vi "Aeroflex ATT Config Test.vi"(8 "error in (no error)":errorcluster, 10 "Configuration":T2={"BusType"=enum."USB", "Card"=0, "USB"="", "IP"=0, "COM"=1, "Baud Rate"=enum."9600"}, 11 "Str Refnum":refnum<vi>) -> (0 "error out":errorcluster, 3 "Aerolex ATT":T1)   [LabVIEW 2011]
uses:
  TypeDefs/Aeroflex ATT Configuration.ctl
  TypeDefs/Aeroflex ATT Instrument Info.ctl
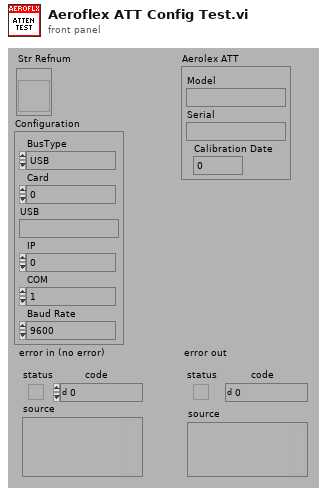
[diagram p1: front panel]
types:
  T1 = typedef "Aeroflex ATT Instrument Info.ctl" = cluster{"Model":string, "Serial":string, "Calibration Date":dbl}
  T2 = typedef "Aeroflex ATT Configuration.ctl" = cluster{"BusType":enum32{"PCI/ISA/PCMCIA", "USB", "Ethernet", "Serial"}, "Card":i32, "USB":string, "IP":u32, "COM":i32, "Baud Rate":enum16{"300", "600", "1200", "2400", "4800", "9600"}}
  T3 = enum32{"PCI/ISA/PCMCIA", "USB", "Ethernet", "Serial"}
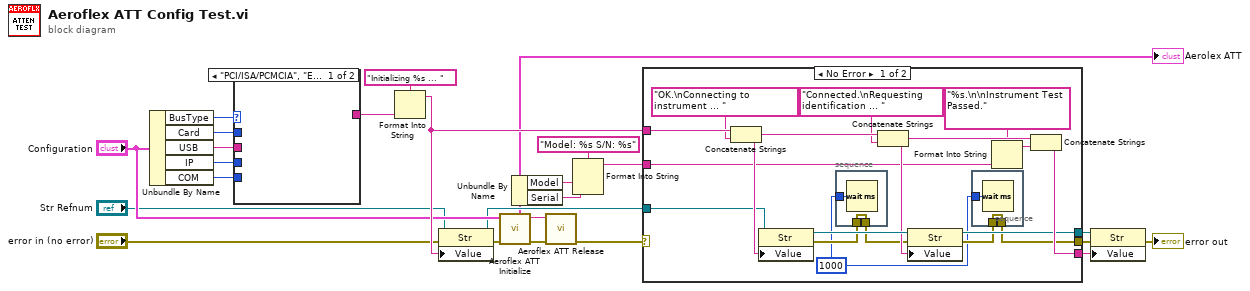
[diagram p0: block diagram]
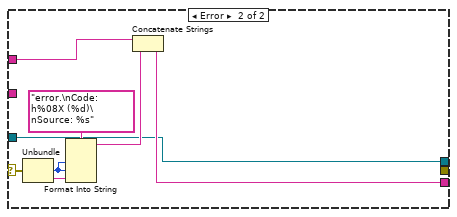
[diagram p2: hidden frame]
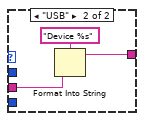
[diagram p3: hidden frame]
diagram:
  n1 = Unbundle By Name("Configuration") -> ("BusType"=w24:T3, "Card"=w23:i32, "USB"=w22:string, "IP"=w21:u32, "COM"=w20:i32)
  n2 = case shown="\"PCI/ISA/PCMCIA\", \"Ethernet\", \"Serial\", Default" w24 {
    tunnel: w23 -> [_ _]
    tunnel: w22 -> [_ w26]
    tunnel: w21 -> [_ _]
    tunnel: w20 -> [_ _]
    tunnel: [_ w27] -> w19
    frame "PCI/ISA/PCMCIA", "Ethernet", "Serial", Default {
    }
    frame "USB" {
      n3 = Format Into String(format string="Device %s", w26) -> (resulting string=w27:string)  [unwired: 2 in, 1 out]
    }
  }
  n4 = Format Into String(format string="Initializing %s ... ", w19) -> (resulting string=w18:string)  [unwired: 2 in, 1 out]
  n5 = property class="Str"(reference="Str Refnum", error in="error in (no error)", "Value"=w18) -> (reference out=w4:refnum<vi>, error out=w16:errorcluster)
  n6 = call "Aeroflex ATT Initialize.vi"("error in (no error)"=w16, "Configuration"="Configuration") -> ("error out"=w14:errorcluster, "DAQmx Dev Name (PAModule)"=w12:string, "Aeroflex ATT"=w1:T1)  [unwired: 7 out]
  "Aerolex ATT" <- w1
  n7 = Unbundle By Name(w1) -> ("Model"=w3:string, "Serial"=w2:string)
  n8 = call "Aeroflex ATT Release.vi"("error in (no error)"=w14, "DAQmx Dev Name (PAModule)"=w12) -> ("error out"=w13:errorcluster)  [unwired: 1 in, 8 out]
  n9 = Format Into String(format string="Model: %s S/N: %s" ("Return Model and Serial #"), w3, w2) -> (resulting string=w11:string)  [unwired: 2 in, 1 out]
  n10 = case shown="No Error" w13 {
    selector: w13 -> [_ w55]
    tunnel: w18 -> [w44 w57]
    tunnel: w4 -> [w39 w50]
    tunnel: w11 -> [w36 _]
    tunnel: [w35 w51] -> w9
    tunnel: [w34 w50] -> w7
    tunnel: [w30 _] -> w6
    frame No Error {
      w29 = u32 1000 ("milliseconds to wait")
      n11 = Concatenate Strings(w44, "OK.\nConnecting to instrument ... ") -> (w42:string)
      n12 = property class="Str"(reference=w39, "Value"=w42) -> (reference out=w45:refnum<vi>, error out=w33:errorcluster)  [unwired: 1 in]
      n13 = stacked-sequence {
        tunnel: w29 -> [w49]
        tunnel: w33 -> [w48]
        tunnel: [w48] -> w32
        frame #0 {
          n14 = Wait (ms)(milliseconds to wait=w49) -> ()  [unwired: 1 out]
        }
      }
      n15 = Concatenate Strings(w42, "Connected.\nRequesting identification ... ") -> (w40:string)
      n16 = property class="Str"(reference=w45, error in=w32, "Value"=w40) -> (reference out=w34:refnum<vi>, error out=w31:errorcluster)
      n17 = stacked-sequence {
        tunnel: w29 -> [w47]
        tunnel: w31 -> [w46]
        tunnel: [w46] -> w30
        frame #0 {
          n18 = Wait (ms)(milliseconds to wait=w47) -> ()  [unwired: 1 out]
        }
      }
      n19 = Format Into String(format string="%s.\n\nInstrument Test Passed.", w36) -> (resulting string=w37:string)  [unwired: 2 in, 1 out]
      n20 = Concatenate Strings(w40, w37) -> (w35:string)
    }
    frame Error {
      n21 = Unbundle(w55) -> ("code"=w54:i32, "source"=w53:string)  [unwired: 1 out]
      n22 = Format Into String(format string="error.\nCode:  h%08X (%d)\nSource: %s", w54, w54, w53) -> (resulting string=w52:string)  [unwired: 2 in, 1 out]
      n23 = Concatenate Strings(w57, w52) -> (w51:string)
    }
  }
  n24 = property class="Str"(reference=w7, error in=w6, "Value"=w9) -> (error out=→"error out":errorcluster)  [unwired: 1 out]
